vi "Format log file to display data.vi"(11 "Master Log":string[][](table)) -> (3 "Formatted table":string[][](table))   [LabVIEW 2011]
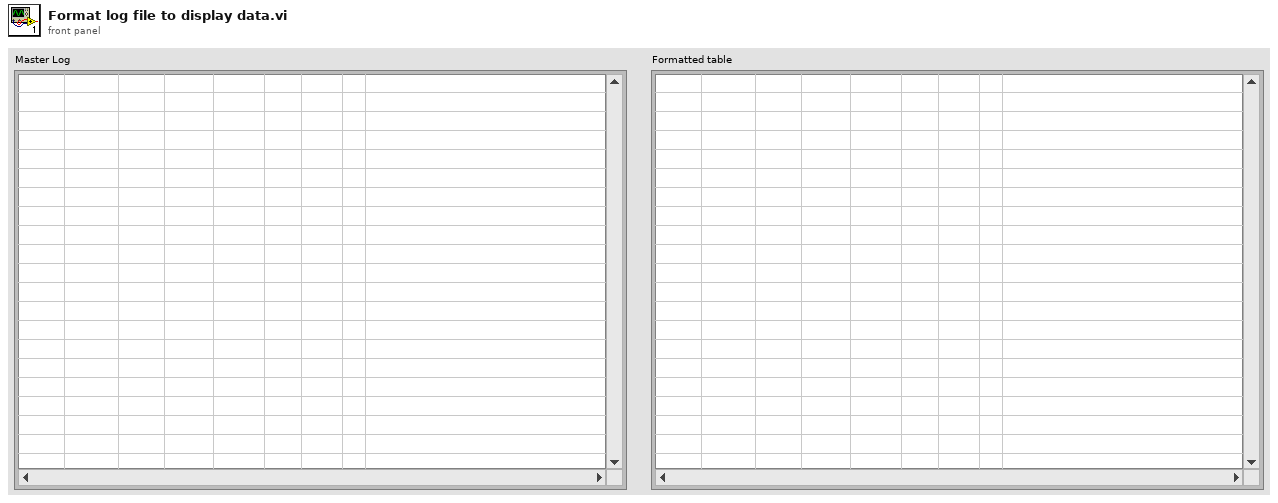
[diagram p1: front panel]
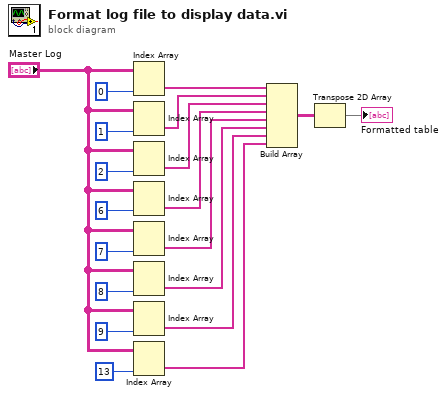
[diagram p0: block diagram]
diagram:
  n1 = Index Array(array="Master Log", index (col)=0) -> (element=w10:string[])  [unwired: 1 in]
  n2 = Index Array(array="Master Log", index (col)=1) -> (element=w9:string[])  [unwired: 1 in]
  n3 = Index Array(array="Master Log", index (col)=2) -> (element=w8:string[])  [unwired: 1 in]
  n4 = Index Array(array="Master Log", index (col)=6) -> (element=w7:string[])  [unwired: 1 in]
  n5 = Index Array(array="Master Log", index (col)=7) -> (element=w6:string[])  [unwired: 1 in]
  n6 = Index Array(array="Master Log", index (col)=8) -> (element=w5:string[])  [unwired: 1 in]
  n7 = Index Array(array="Master Log", index (col)=9) -> (element=w4:string[])  [unwired: 1 in]
  n8 = Index Array(array="Master Log", index (col)=13) -> (element=w3:string[])  [unwired: 1 in]
  n9 = Build Array(w10, w9, w8, w7, w6, w5, w4, w3) -> (w2:string[][])
  n10 = Transpose 2D Array(2D array=w2) -> (transposed array=→"Formatted table":string[][])
